vi "get move settings.vi"(8 "error in (no error)":errorcluster, 10 "move_settings":T1, 11 "id":i32) -> (0 "error out":errorcluster, 2 "move_settings out":T1, 3 "function return":i32)   [LabVIEW 2012, in "libximc.lvlib"]
doc: "result_t XIMC_API get_move_settings (device_t id, move_settings_t* move_settings);"
uses:
  libximc.lvlib
  libximc.dll
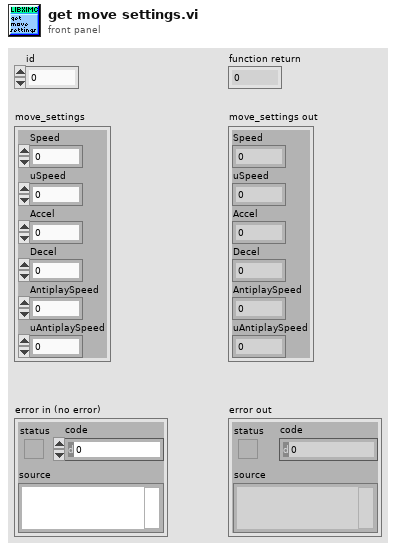
[diagram p1: front panel]
types:
  T1 = cluster{"Speed":u32, "uSpeed":u32, "Accel":u32, "Decel":u32, "AntiplaySpeed":u32, "uAntiplaySpeed":u32}
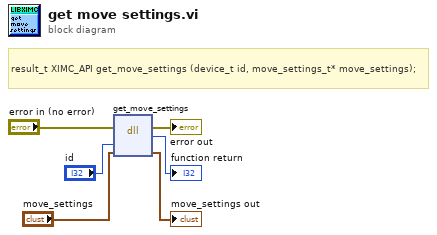
[diagram p0: block diagram]
diagram:
  # "result_t XIMC_API get_move_settings (device_t id, move_settings_t* move_settings);"
  n1 = dll-call lib="E:/labview-2.12.1-Labview_12.0/ximcLVx32/libximc.*" fn="get_move_settings"(error in="error in (no error)", "id"="id", "move_settings"="move_settings") -> (error out=→"error out":errorcluster, →"function return":i32, "move_settings"=→"move_settings out":T1)  [unwired: 3 in, 1 out]
